vi "VelocityCommand1D.vi"(4 "PID gains Vel D":cluster{"(Kp)":dbl, "(Ki)":dbl, "(Kd)":dbl}, 5 "output xy":dbl format="%#_13g", 6 "intervalo":dbl, 7 "size error array":i32, 9 "est_v":dbl, 10 "Velocities":dbl[](array[numeric]), 11 "Time":dbl[](array[numeric])) -> (3 "uk":dbl)   [LabVIEW 2018]
uses:
  <vilib>/Analysis/baseanly.llb/Real Dot Product.vi
  <vilib>/Analysis/NI_AALBase.lvlib
panel:
  out "Waveform Chart":cluster{dbl, dbl, dbl, dbl}(graph)
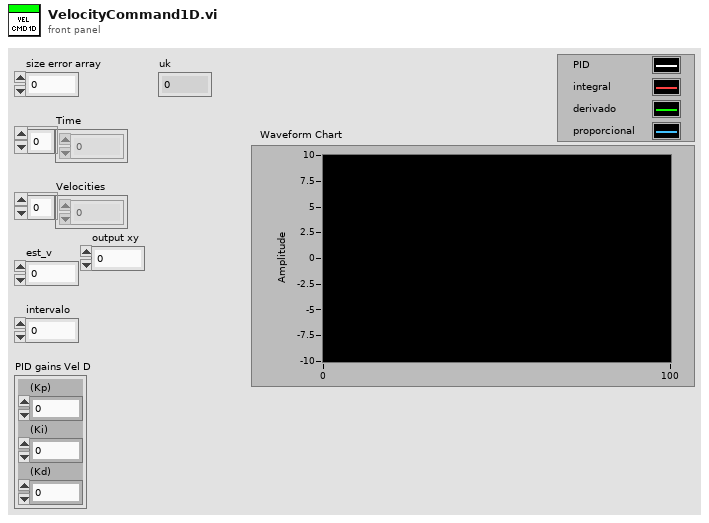
[diagram p1: front panel]
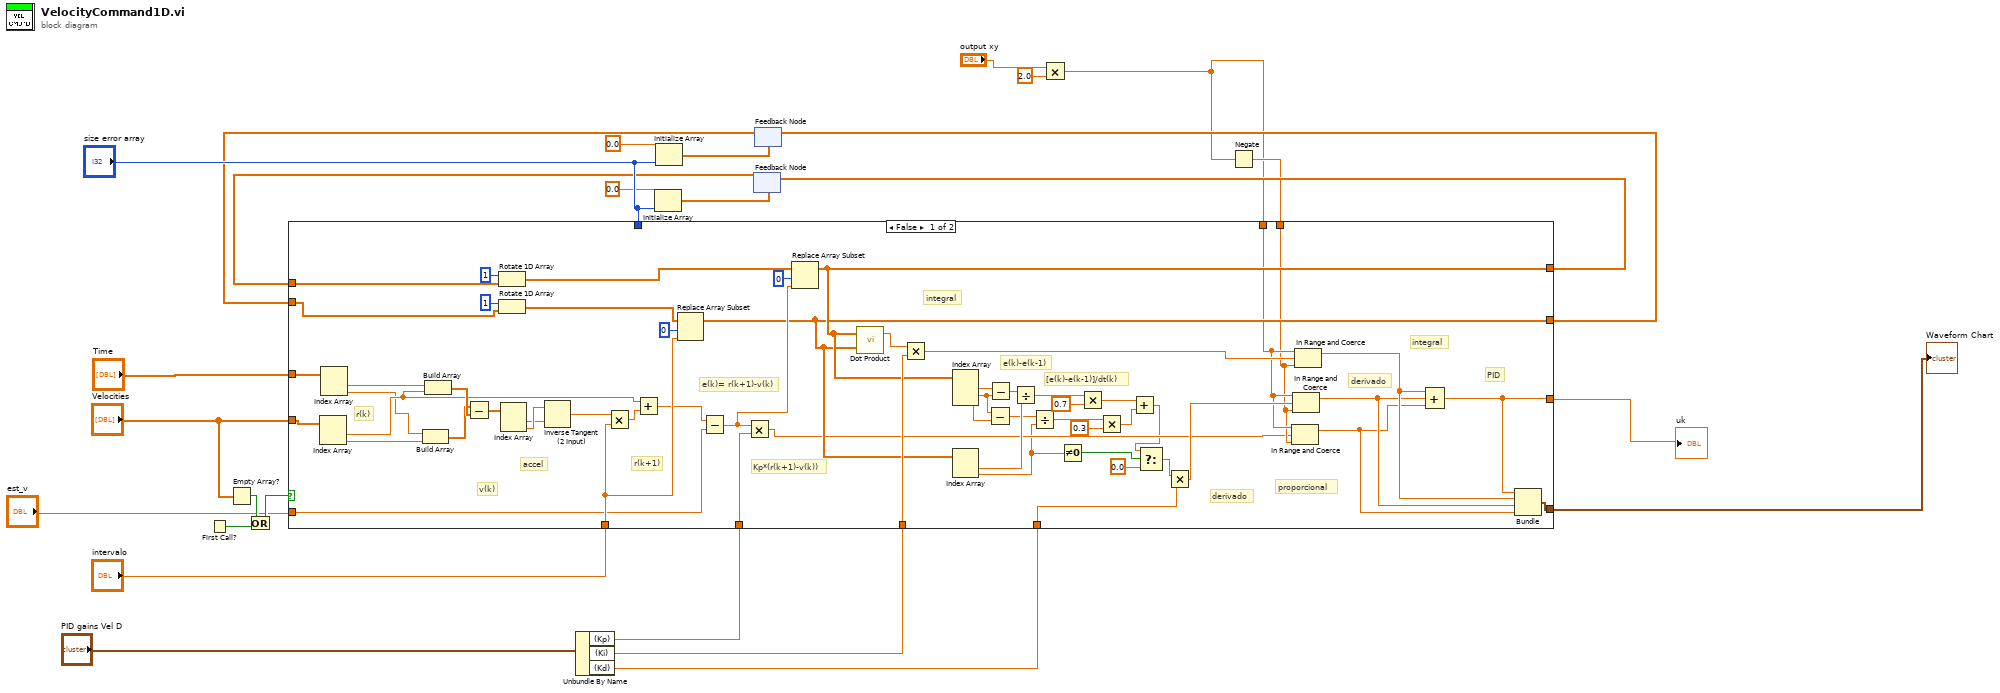
[diagram p0: block diagram]
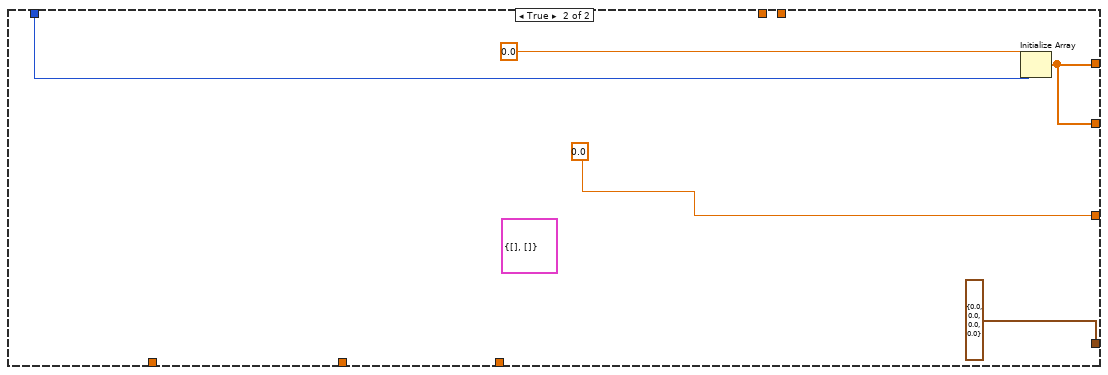
[diagram p2: hidden frame]
diagram:
  n1 = First Call?() -> (First Call?: T/F=w15:bool)
  n2 = Empty Array?(array="Velocities") -> (empty?=w14:bool)
  n3 = Or(x=w14, y=w15) -> (x .or. y?=w16:bool)
  n4 = Unbundle By Name("PID gains Vel D") -> ("(Kp)"=w23:dbl, "(Ki)"=w24:dbl, "(Kd)"=w25:dbl)
  n5 = Initialize Array(0.0 ("element"), "size error array") -> (w8:dbl[])
  n6 = Initialize Array(0.0 ("element"), "size error array") -> (w19:dbl[])
  n7 = feedback #1(w8) -> (w10:dbl[])
  n8 = feedback #2(w19) -> (w20:dbl[])
  n9 = Multiply(x="output xy", y=2.0) -> (x*y=w3:dbl)
  n10 = Negate(x=w3) -> (-x=w5:dbl)
  n11 = case shown="False" w16 {
    tunnel: "intervalo" -> [w66 _]
    tunnel: "Time" -> [w84 _]
    tunnel: [w43 0.0 ("v3")] -> w17
    tunnel: "Velocities" -> [w83 _]
    tunnel: w10 -> [w75 _]
    tunnel: [w58 w87] -> w11
    tunnel: "est_v" -> [w63 _]
    tunnel: w20 -> [w68 _]
    tunnel: [w56 w87] -> w21
    tunnel: w23 -> [w62 _]
    tunnel: w24 -> [w59 _]
    tunnel: w25 -> [w41 _]
    tunnel: "size error array" -> [_ w86]
    tunnel: w3 -> [w50 _]
    tunnel: w5 -> [w49 _]
    tunnel: [w47 cluster{dbl, dbl, dbl, dbl} {0.0, 0.0, 0.0, 0.0} ("Cluster 2")] -> w1
    frame False {
      # "PID"
      # "proporcional"
      # "derivado"
      # "integral"
      # "r(k)"
      # "derivado"
      # "[e(k)-e(k-1)]/dt(k)"
      # "e(k)-e(k-1)"
      # "integral"
      # "Kp*(r(k+1)-v(k))"
      # "e(k)= r(k+1)-v(k)"
      # "v(k)"
      # "r(k+1)"
      # "accel"
      n12 = Index Array(array=w83) -> (element #1=w65:dbl, element #2=w76:dbl)  [unwired: 2 in]
      n13 = Index Array(array=w84) -> (element #1=w46:dbl, element #2=w64:dbl)  [unwired: 2 in]
      n14 = Build Array(w64, w76) -> (w81:dbl[])
      n15 = Build Array(w46, w65) -> (w82:dbl[])
      n16 = Subtract(x=w81, y=w82) -> (x-y=w80:dbl[])
      n17 = Rotate 1D Array(1:w75, 2:1 ("n")) -> (0:w73:dbl[])
      n18 = Rotate 1D Array(1:w68, 2:1 ("n")) -> (0:w67:dbl[])
      n19 = Index Array(array=w80) -> (element #1=w78:dbl, element #2=w79:dbl)  [unwired: 2 in]
      n20 = Inverse Tangent (2 Input)(1:w78, 2:w79) -> (0:w77:dbl)
      n21 = Multiply(x=w77, y=w66) -> (x*y=w71:dbl)
      n22 = Add(x=w65, y=w71) -> (x+y=w53:dbl)
      n23 = Replace Array Subset(array=w67, new element=w66, index=0) -> (w56:dbl[])
      n24 = Subtract(x=w53, y=w63) -> (x-y=w61:dbl)
      n25 = Multiply(x=w61, y=w62) -> (x*y=w48:dbl)
      n26 = Replace Array Subset(array=w73, new element=w61, index=0) -> (w58:dbl[])
      n27 = call-poly <vilib>:"Dot Product.vi"("Y Vector"=w56, "X Vector"=w58) -> ("X * Y"=w60:dbl)  [unwired: 1 out]
      n28 = Multiply(x=w60, y=w59) -> (x*y=w52:dbl)
      n29 = Index Array(array=w58) -> (element #1=w57:dbl, element #2=w40:dbl, element #3=w39:dbl)  [unwired: 3 in]
      n30 = Index Array(array=w56) -> (element #1=w54:dbl, element #2=w28:dbl)  [unwired: 2 in]
      n31 = Subtract(x=w40, y=w39) -> (x-y=w38:dbl)
      n32 = Subtract(x=w57, y=w40) -> (x-y=w55:dbl)
      n33 = Divide(x=w55, y=w54) -> (x/y=w37:dbl)
      n34 = Divide(x=w38, y=w28) -> (x/y=w34:dbl)
      n35 = Not Equal To 0?(x=w28) -> (x != 0?=w27:bool)
      n36 = Multiply(x=w37, y=0.7) -> (x*y=w32:dbl)
      n37 = Multiply(x=w34, y=0.3) -> (x*y=w33:dbl)
      n38 = Add(x=w32, y=w33) -> (x+y=w30:dbl)
      n39 = Select(t=w30, s=w27, f=0.0) -> (s? t:f=w31:dbl)
      n40 = Multiply(x=w31, y=w41) -> (x*y=w51:dbl)
      n41 = In Range and Coerce(upper limit=w50, x=w48, lower limit=w49) -> (coerced(x)=w42:dbl)  [unwired: 1 out]
      n42 = In Range and Coerce(upper limit=w50, x=w51, lower limit=w49) -> (coerced(x)=w44:dbl)  [unwired: 1 out]
      n43 = In Range and Coerce(upper limit=w50, x=w52, lower limit=w49) -> (coerced(x)=w45:dbl)  [unwired: 1 out]
      n44 = Compound Arithmetic op=ADD(w45, w44, w42) -> (w43:dbl)
      n45 = Bundle(w43, w45, w44, w42) -> (w47:cluster{dbl, dbl, dbl, dbl})  [unwired: 1 in]
    }
    frame True {
      (unwired) cluster{dbl[], dbl[]} {[], []} ("Cluster")
      n46 = Initialize Array(0.0 ("element"), w86) -> (w87:dbl[])
    }
  }
  "uk" <- w17
  "Waveform Chart" <- w1
  n47 = feedback-in #1(w11) -> ()
  n48 = feedback-in #2(w21) -> ()
